vi "VMI_save_Files.vi"(1 "Peaks":T2[](array[typedef]), 2 "Save":bool[](array[boolean]), 3 "Image Info":T1={"X size"=782.0, "Y size"=582.0, "Centroiding"=1.0}, 4 "Hist_full":dbl[][][](array[numeric]), 5 "Current File Date":string, 6 "error in (no error)":errorcluster, 7 "Collection Information":T3[](array[typedef]), 8 "ChangeFile":bool, 9 "Histogram_array":i32[][](array[numeric]), 10 "appended path":path=path "C:/Users/Parkes/Documents/GitHub/Camera-Acquire_Labview/120416aa") -> (0 "error out":errorcluster)   [LabVIEW 2018]
uses:
  Type defs/FileAcq_v1_Ctrl.ctl
  Type defs/VMI_peak_out.ctl
  Type defs/Image_info.ctl
  Type defs/Header_infor_IF32.ctl
  <vilib>/Utility/file.llb/Write Delimited Spreadsheet (string).vi
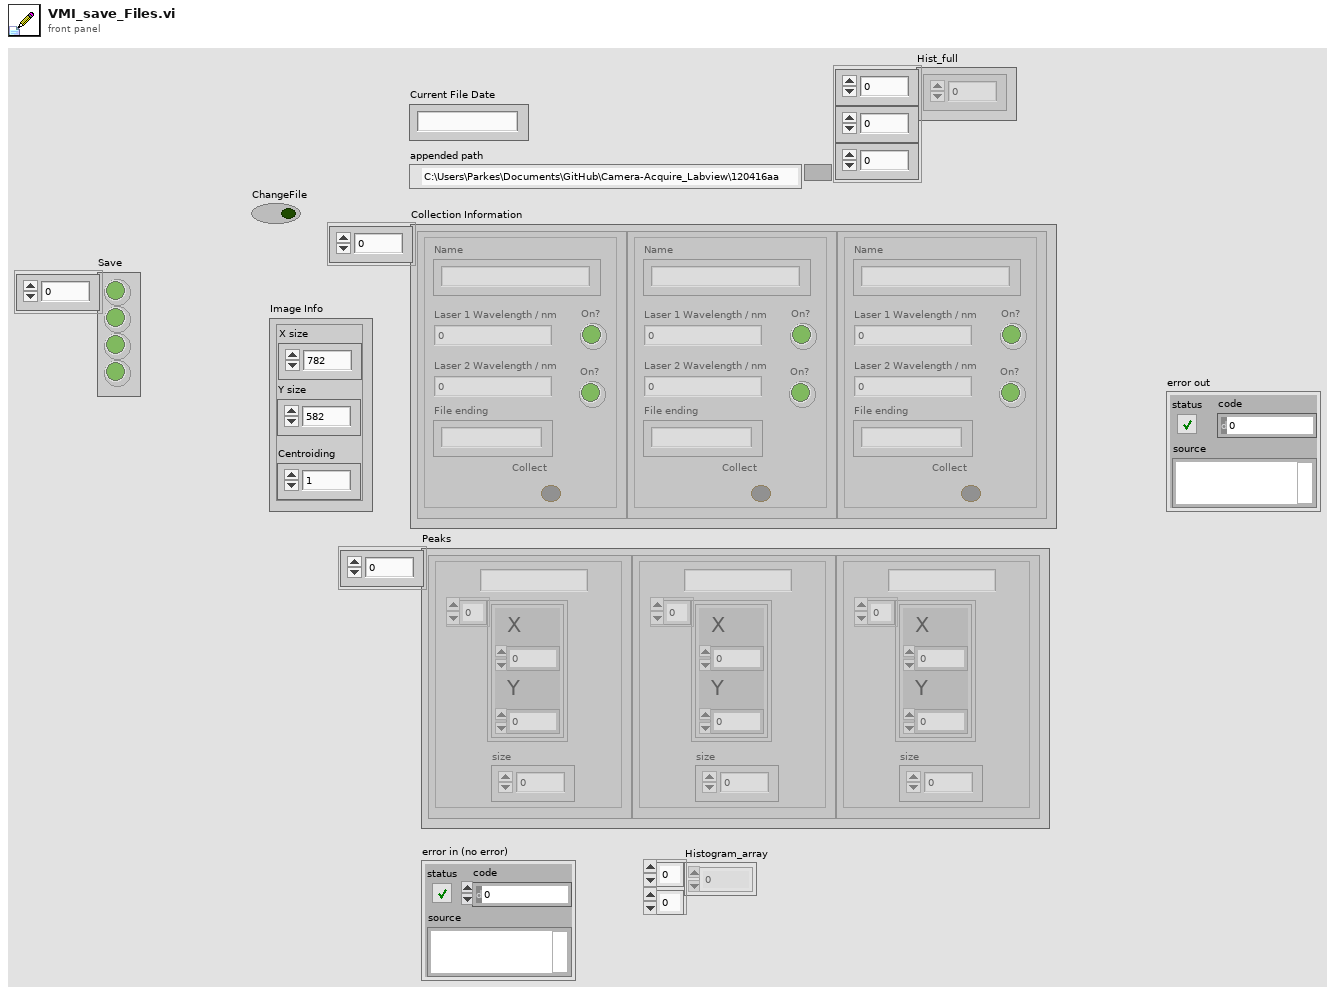
[diagram p1: front panel]
types:
  T1 = typedef "Image_info.ctl" = cluster{"X size":dbl, "Y size":dbl, "Centroiding":dbl}
  T2 = typedef "VMI_peak_out.ctl" = cluster{"Peaks":cluster{"X":sgl, "Y":sgl}[], "size":i32, "Title":string}
  T3 = typedef "FileAcq_v1_Ctrl.ctl" = cluster{"Type":string, "LaserWave1":dbl, "Shutter1":bool, "LaserWave2":dbl, "Shutter2":bool, "FileEnd":string, "Collect":bool}
  T4 = typedef "Header_infor_IF32.ctl" = cluster{"File Name":string, "Time":string, "Date":string, "Size":string}
  T5 = enum16{"open", "replace", "create", "open or create", "replace or create", "replace or create with confirmation"}
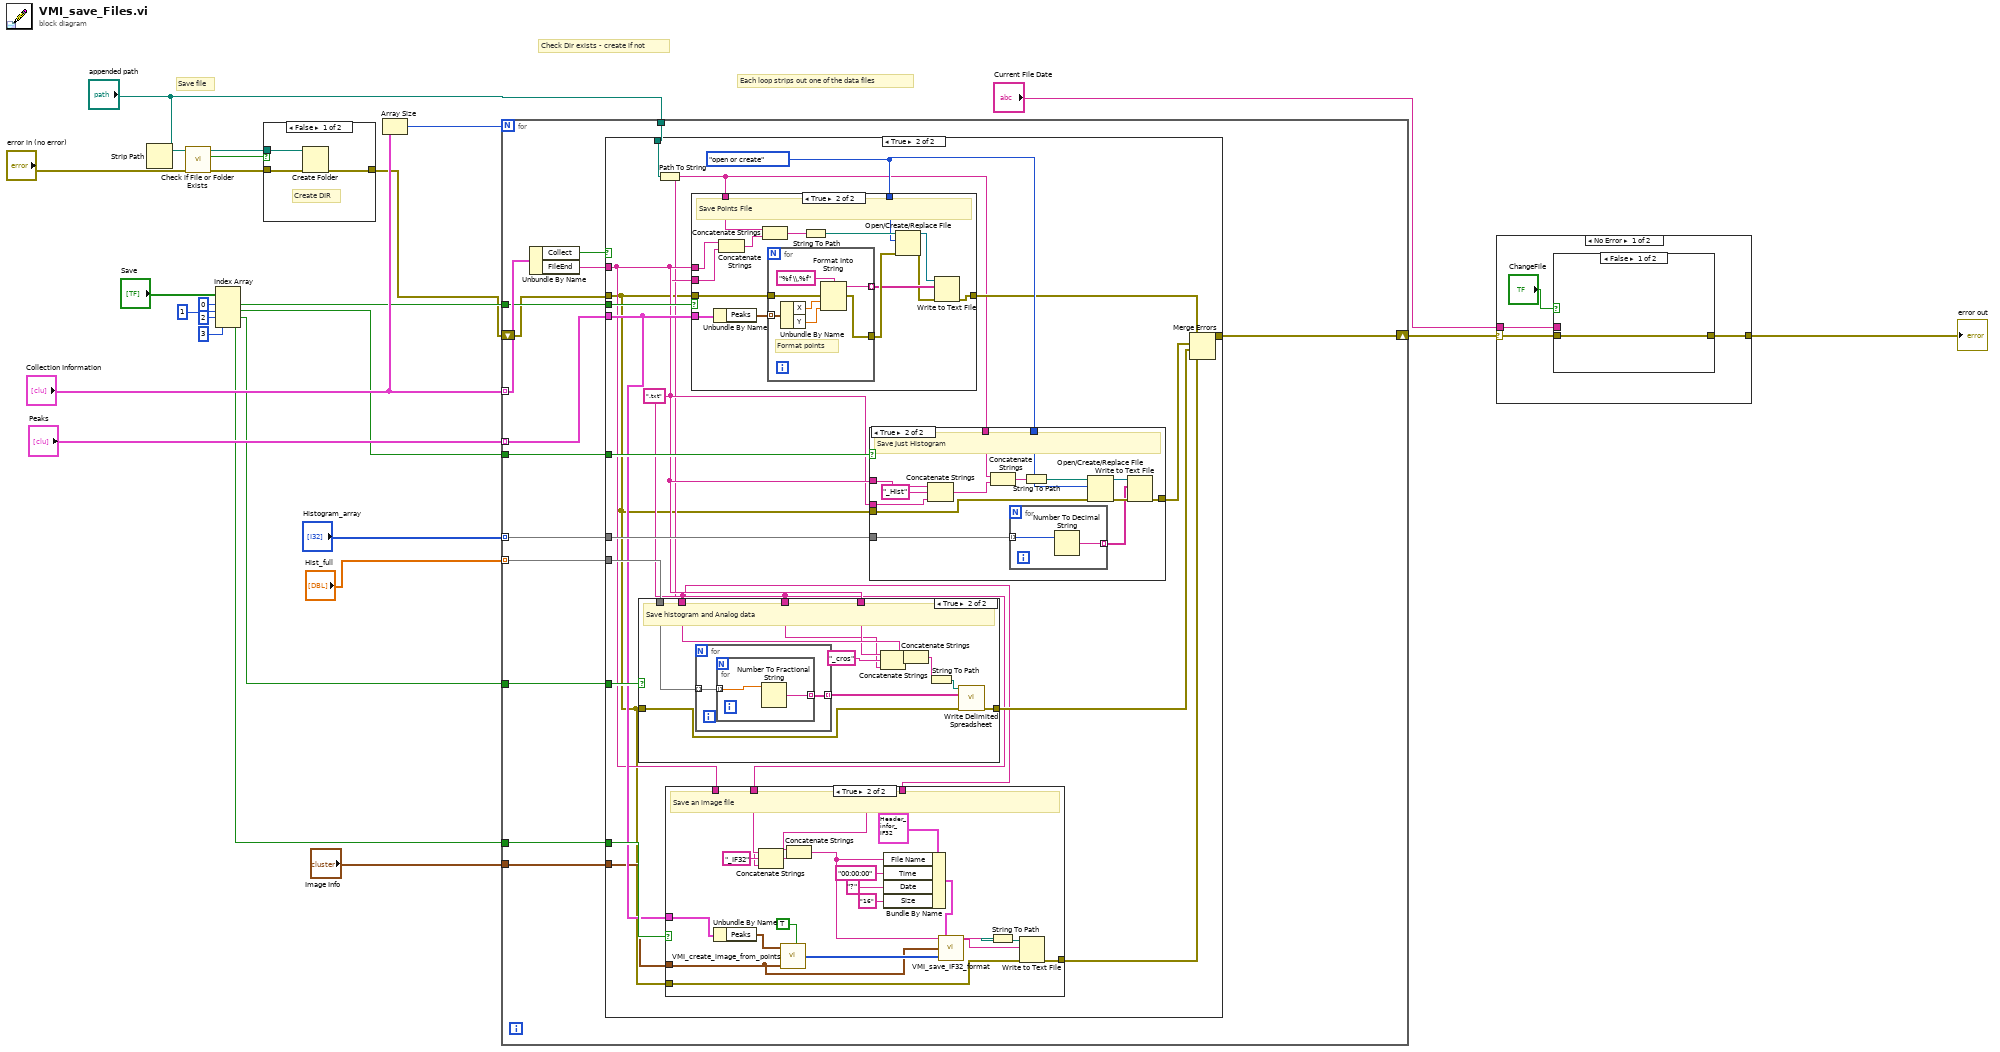
[diagram p0: block diagram]
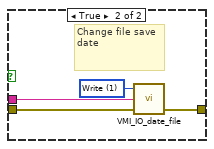
[diagram p2: hidden frame]
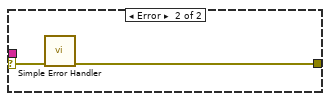
[diagram p3: hidden frame]
diagram:
  # "Each loop strips out one of the data files"
  # "Check Dir exists - create if not"
  # "Save file"
  n1 = Strip Path(path="appended path") -> (stripped path=w23:path)  [unwired: 1 out]
  n2 = call <vilib>:"Check if File or Folder Exists.vi"("error in (no error)"="error in (no error)", "path"=w23) -> ("error out"=w20:errorcluster, "file or folder exists?"=w22:bool, "dup path"=w21:path)  [unwired: 7 in]
  n3 = Index Array(array="Save", index #1=0 ("index"), index #2=1 ("index"), index #3=2 ("index"), index #4=3 ("index")) -> (element #1=w9:bool, element #2=w7:bool, element #3=w8:bool, element #4=w5:bool)
  n4 = case shown="False" w22 {
    tunnel: w21 -> [w27 _]
    tunnel: w20 -> [w26 w28]
    tunnel: [w25 w28] -> w3
    frame False {
      # "Create DIR"
      n5 = Create Folder(path (use dialog)=w27, error in=w26) -> (error out=w25:errorcluster)  [unwired: 1 in, 2 out]
    }
    frame True {
    }
  }
  n6 = Array Size(array="Collection Information") -> (size(s)=w17:i32)
  n7 = for {
    N: w17 -> [_]
    tunnel: "Collection Information" -> [w40] mode=indexing
    tunnel: "appended path" -> [w42]
    tunnel: "Histogram_array" -> [w41] mode=indexing
    tunnel: "Peaks" -> [w36] mode=indexing
    tunnel: "Hist_full" -> [w37] mode=indexing
    tunnel: w9 -> [w35]
    tunnel: w8 -> [w34]
    tunnel: w7 -> [w33]
    tunnel: w5 -> [w32]
    tunnel: "Image Info" -> [w31]
    shift-right: [w29] -> w2
    shift-left: w3 -> [w30]
    n8 = Unbundle By Name(w40) -> ("Collect"=w39:bool, "FileEnd"=w38:string)
    n9 = case shown="True" w39 {
      tunnel: w42 -> [_ w62]
      tunnel: [w43 w59] -> w29
      tunnel: w30 -> [w43 w45]
      tunnel: w41 -> [_ w61]
      tunnel: w38 -> [_ w48]
      tunnel: w37 -> [_ w58]
      tunnel: w36 -> [_ w50]
      tunnel: w35 -> [_ w53]
      tunnel: w34 -> [_ w54]
      tunnel: w33 -> [_ w52]
      tunnel: w32 -> [_ w51]
      tunnel: w31 -> [_ w49]
      frame False {
      }
      frame True {
        w56 = T5."open or create" ("operation (0:open)")
        w47 = ".txt" ("string")
        n10 = Path To String(path=w62) -> (string=w46:string)
        n11 = case shown="True" w54 {
          tunnel: w58 -> [_ w112]
          tunnel: [w101 w106] -> w57
          tunnel: w46 -> [_ w105]
          tunnel: w48 -> [_ w104]
          tunnel: w45 -> [w101 w102]
          tunnel: w47 -> [_ w103]
          frame False {
          }
          frame True {
            # "Save histogram and Analog data"
            n12 = for {
              tunnel: w112 -> [w114] mode=indexing
              tunnel: [w113] -> w111 mode=indexing
              n13 = for {
                tunnel: w114 -> [w116] mode=indexing
                tunnel: [w115] -> w113 mode=indexing
                n14 = Number To Fractional String(number=w116) -> (F-format string=w115:string)  [unwired: 3 in]
              }
            }
            n15 = Concatenate Strings(w104, "_cros" ("string"), w103) -> (w109:string)
            n16 = Concatenate Strings(w105, w109) -> (w108:string)
            n17 = String To Path(string=w108) -> (path=w107:path)
            n18 = call-poly <vilib>:"Write Delimited Spreadsheet.vi"("file path (dialog if empty)"=w107, "2D data"=w111, "error in (no error)"=w102) -> ("error out"=w106:errorcluster)  [unwired: 11 in, 1 out]
          }
        }
        n19 = case shown="True" w51 {
          tunnel: w50 -> [_ w82]
          tunnel: w49 -> [_ w79]
          tunnel: w48 -> [_ w78]
          tunnel: w47 -> [_ w76]
          tunnel: w46 -> [_ w74]
          tunnel: w45 -> [w63 w71]
          tunnel: [w63 w70] -> w44
          frame False {
          }
          frame True {
            # "Save an image file"
            n20 = Unbundle By Name(w82) -> ("Peaks"=w81:cluster{"X":sgl, "Y":sgl}[])
            n21 = Concatenate Strings(w78, "_IF32" ("string"), w76) -> (w75:string)
            n22 = call "VMI_create_image_from_points.vi"("New Array"=TRUE, "Image Info"=w79, "Points"=w81) -> ("Image Array"=w80:i16[][])  [unwired: 2 in]
            n23 = Concatenate Strings(w74, w75) -> (w64:string)
            n24 = Bundle By Name(cluster=T4 {"File Name"="080916aa", "Time"="Hammer", "Date"="Now", "Size"=""} ("Cluster"), "File Name"=w64, "Time"="00:00:00", "Date"="?", "Size"="16") -> (w65:T4)
            n25 = call "VMI_save_IF32_format.vi"("Image Array"=w80, "Image Info"=w79, "Header Cluster"=w65) -> ("File String"=w72:string)  [unwired: 2 in]
            n26 = String To Path(string=w64) -> (path=w73:path)
            n27 = Write to Text File(file (use dialog)=w73, text=w72, error in=w71) -> (error out=w70:errorcluster)  [unwired: 1 in, 2 out]
          }
        }
        n28 = case shown="True" w53 {
          tunnel: [w117 w118] -> w55
          tunnel: w45 -> [w117 w132]
          tunnel: w47 -> [_ w131]
          tunnel: w48 -> [_ w130]
          tunnel: w50 -> [_ w129]
          tunnel: w46 -> [_ w127]
          tunnel: w56 -> [_ w122]
          frame False {
          }
          frame True {
            # "Save Points File"
            n29 = Unbundle By Name(w129) -> ("Peaks"=w128:cluster{"X":sgl, "Y":sgl}[])
            n30 = Concatenate Strings(w130, w131) -> (w126:string)
            n31 = Concatenate Strings(w127, w126) -> (w125:string)
            n32 = for {
              tunnel: w128 -> [w139] mode=indexing
              tunnel: [w135] -> w120 mode=indexing
              tunnel: [w134] -> w123
              tunnel: w132 -> [w133]
              # "Format points"
              n33 = Unbundle By Name(w139) -> ("X"=w138:sgl, "Y"=w137:sgl)
              n34 = Format Into String(format string="%f \\,%f", error in=w133, w138, w137) -> (resulting string=w135:string, error out=w134:errorcluster)  [unwired: 1 in]
            }
            n35 = String To Path(string=w125) -> (path=w124:path)
            n36 = Open/Create/Replace File(file path (use dialog)=w124, error in=w123, operation (0:open)=w122) -> (refnum out=w121:refnum<file>, error out=w119:errorcluster)  [unwired: 3 in, 1 out]
            n37 = Write to Text File(file (use dialog)=w121, text=w120, error in=w119) -> (error out=w118:errorcluster)  [unwired: 1 in, 2 out]
          }
        }
        n38 = case shown="True" w52 {
          tunnel: w47 -> [_ w97]
          tunnel: w61 -> [_ w91]
          tunnel: [w84 w89] -> w60
          tunnel: w46 -> [_ w88]
          tunnel: w56 -> [_ w87]
          tunnel: w48 -> [_ w86]
          tunnel: w45 -> [w84 w85]
          frame False {
          }
          frame True {
            # "Save Just Histogram"
            n39 = Concatenate Strings(w86, "_Hist" ("string"), w97) -> (w96:string)
            n40 = Concatenate Strings(w88, w96) -> (w95:string)
            n41 = for {
              tunnel: w91 -> [w100] mode=indexing
              tunnel: [w99] -> w90 mode=indexing
              n42 = Number To Decimal String(number=w100) -> (decimal integer string=w99:string)  [unwired: 1 in]
            }
            n43 = String To Path(string=w95) -> (path=w94:path)
            n44 = Open/Create/Replace File(file path (use dialog)=w94, error in=w85, operation (0:open)=w87) -> (refnum out=w93:refnum<file>, error out=w92:errorcluster)  [unwired: 3 in, 1 out]
            n45 = Write to Text File(file (use dialog)=w93, text=w90, error in=w92) -> (error out=w89:errorcluster)  [unwired: 1 in, 2 out]
          }
        }
        n46 = Merge Errors(w55, w60, w57, w44) -> (w59:errorcluster)
      }
    }
  }
  "error out" <- w2
  n47 = case shown="No Error" w2 {
    selector: w2 -> [w142 w150]
    tunnel: "Current File Date" -> [w143 _]
    tunnel: [w141 w149] -> _
    frame No Error {
      n48 = case shown="False" "ChangeFile" {
        tunnel: w143 -> [_ w148]
        tunnel: w142 -> [w144 w147]
        tunnel: [w144 w145] -> w141
        frame False {
        }
        frame True {
          w146 = u16 1 items=["Read", "Write"] ("File Task")
          # "Change file save\ndate"
          n49 = call "VMI_IO_date_file.vi"("Error In"=w147, "File date in"=w148, "File Task"=w146) -> ("Error Out"=w145:errorcluster)  [unwired: 1 in, 1 out]
        }
      }
    }
    frame Error {
      n50 = call <vilib>:"Simple Error Handler.vi"("error in (no error)"=w150) -> ("error out"=w149:errorcluster)  [unwired: 4 in, 4 out]
    }
  }
